vi "XYStage.ReadVelocity.vi"(8 "error in (no error)":errorcluster, 11 "XYStage in":refnum<class "XYStage.lvclass">) -> (0 "error out":errorcluster, 1 "Velocity (counts/s)":i32, 2 "Velocity (units/s)":dbl, 3 "XYStage out":refnum<class "XYStage.lvclass">)   [LabVIEW 2015, in "XYStage.lvclass"]
uses:
  XYStage.lvclass
  XYStage.lvclass/XYStage.ctl
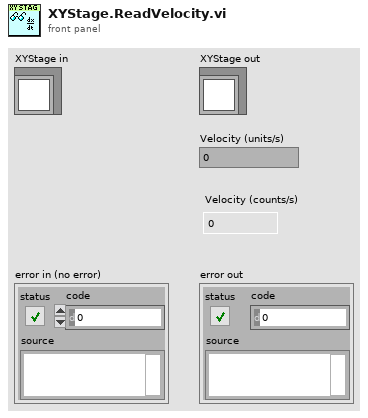
[diagram p1: front panel]
types:
  T1 = typedef "XYStage.lvclass/PrivateData--Ref.ctl" = refnum<data-value>
  T2 = typedef "XYStage.lvclass/PrivateData--Cluster.ctl" = cluster{"Dependencies":T3, "Public Events":T4, "Protected Events":T5, "Private Events":T6, "Configuration":T7, "Target":T8, "Move Parameters":T11}
  T3 = typedef "XYStage.lvclass/Dependencies--Cluster.ctl" = cluster{"Positions":refnum<class "SMO.Dictionary.Variant.lvclass">}
  T4 = typedef "XYStage.lvclass/PublicEvents--Cluster.ctl" = cluster{"MoveComplete":refnum<user-event>, "NewPosition":refnum<user-event>, "UpdatedNamedPosition":refnum<user-event>, "MoveStarted":refnum<user-event>}
  T5 = typedef "XYStage.lvclass/ProtectedEvents--Cluster.ctl" = cluster{"API_Template":refnum<user-event>}
  T6 = typedef "XYStage.lvclass/PrivateEvents--Cluster.ctl" = cluster{"MoveAbsolute":refnum<user-event>, "MoveRelative":refnum<user-event>, "MoveToNamedPosition":refnum<user-event>, "StorePosition":refnum<user-event>, "Home":refnum<user-event>}
  T7 = typedef "XYStage.lvclass/Configuration--Cluster.ctl" = cluster{"Real-World Units":string, "Counts per Unit":dbl}
  T8 = typedef "XYStage.lvclass/TargetPositions--Cluster.ctl" = cluster{"Coords":T9, "Counts":T10}
  T9 = typedef "XYStage.lvclass/(real)Coords--Cluster.ctl" = cluster{"X":dbl, "Y":dbl}
  T10 = typedef "XYStage.lvclass/(counts)Coords--Cluster.ctl" = cluster{"X":i32, "Y":i32}
  T11 = typedef "XYStage.lvclass/MoveParameters--Cluster.ctl" = cluster{"Velocity (units/s)":dbl, "Acceleration (units/s^2)":dbl}
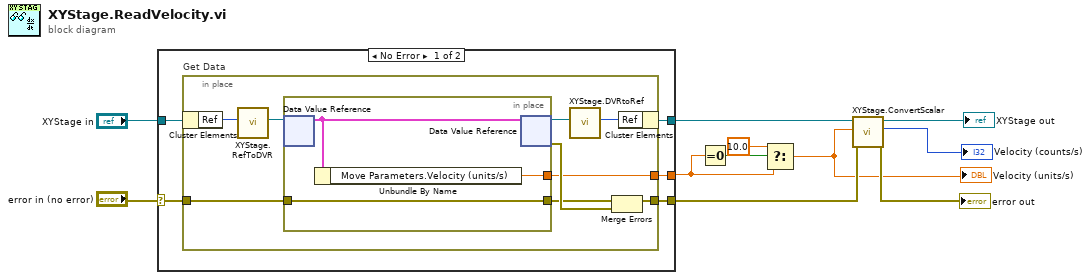
[diagram p0: block diagram]
diagram:
  n1 = case shown="No Error" "error in (no error)" {
    selector: "error in (no error)" -> [w15 w29]
    tunnel: "XYStage in" -> [w16 w30]
    tunnel: [w13 w29] -> w8
    tunnel: [w14 w30] -> w6
    tunnel: [w12 _] -> w3
    frame No Error {
      n2 = in-place "Get Data" {
        in-place-border: w15 -> [w25]
        in-place-border: [w22] -> w13
        in-place-border: [w21] -> w12
        n3 = in-place-cluster #1(w16) -> ("Ref"=w20:u32)
        n4 = call "XYStage.RefToDVR.vi"("Ref"=w20) -> ("Ref"=w18:T1)  [unwired: 10 in]
        n5 = in-place {
          in-place-border: w25 -> [w27]
          in-place-border: [w27] -> w23
          in-place-border: [w26] -> w21
          n6 = in-place-dvr #2(w18) -> (w28:T2)  [unwired: 1 out]
          n7 = Unbundle By Name(w28) -> ("Move Parameters.Velocity (units/s)"=w26:dbl)
          n8 = in-place-dvr #2(w28) -> (w19:T1, w24:errorcluster)
        }
        n9 = call "XYStage.DVRtoRef.vi"("Ref"=w19) -> ("Ref"=w17:u32)  [unwired: 10 in]
        n10 = Merge Errors(w23, w24) -> (w22:errorcluster)
        n11 = in-place-cluster #1("Ref"=w17) -> (w14:refnum<class "XYStage.lvclass">)
      }
    }
    frame Error {
    }
  }
  n12 = Equal To 0?(x=w3) -> (x = 0?=w4:bool)
  n13 = Select(t=10.0, s=w4, f=w3) -> (s? t:f=w2:dbl)
  "Velocity (units/s)" <- w2
  n14 = call-dynamic "XYStage.ConvertScalar.vi"("error in (no error)"=w8, "Units"=w2, "XYStage in"=w6) -> ("error out"=→"error out":errorcluster, "Counts out"=→"Velocity (counts/s)":i32, "XYStage out"=→"XYStage out":refnum<class "XYStage.lvclass">)  [unwired: 5 in, 1 out]
